vi "main.vi"() -> ()   [LabVIEW 2018]
uses:
  <vilib>/Platform/TimedLoop/XDataNode/XDataNode.xnode
  <vilib>/Platform/TimedLoop/XDataNode/nitl_modes.ctl
  <vilib>/Platform/TimedLoop/XDataNode/XDNodeRunTimeDep.lvlib
  <vilib>/Platform/TimedLoop/XDataNode/wakeup.ctl
  <vilib>/Platform/TimedLoop/XDataNode/timing_clust.ctl
  <vilib>/rvi/interface/nirviOpenFPGA/nirviOpenFPGA.xnode
  <vilib>/rvi/interface/nirviReadWriteControl/nirviReadWriteControl.xnode
  <vilib>/rvi/interface/Simulation/niFpgaSimulationCallBeginRW.vi
  <vilib>/rvi/errors/niLvFpgaAdjustHostInterfaceError.vi
  Labview_code/control6acater01.vi
  NiFpgaLv.dll
  <vilib>/Utility/error.llb/Error Cluster From Error Code.vi
  FPGA Bitfiles/Control 1.ctl
panel:
  out "Input Command":dbl[](array[numeric])
  out "now pwm":T1
  out "Finished delay inner loop":i32
  out "notEndmission":bool
  out "Finished delay":i32
  out "Good solution":bool
  out "length of each link":T2
  out "output PWM":cluster{dbl, dbl, dbl, dbl, dbl, dbl}
  in  "stop":T3
  # "StewHoward Platform"
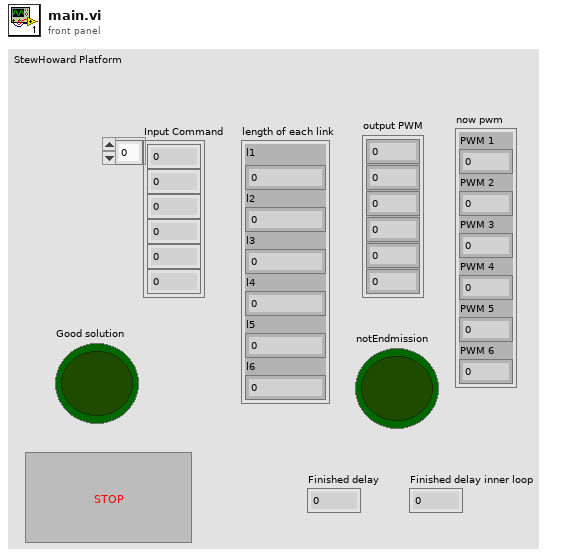
[diagram p1: front panel]
types:
  T1 = cluster{"PWM 1":dbl, "PWM 2":dbl, "PWM 3":dbl, "PWM 4":dbl, "PWM 5":dbl, "PWM 6":dbl}
  T2 = cluster{"l1":dbl, "l2":dbl, "l3":dbl, "l4":dbl, "l5":dbl, "l6":dbl}
  T3 = typedef "Control 1.ctl" = bool
  T4 = typedef "XDNodeRunTimeDep.lvlib/timing_clust.ctl" = cluster{"Expected End [f-1]":u64, "Actual End [f-1]":u64, "Finished Late? [f-1]":bool, "Expected End [i-1]":u64, "Actual End [i-1]":u64, "Finished Late? [i-1]":bool, "Expected Start [i]":u64, "Actual Start [i]":u64, "Expected Start [f]":u64, "Actual Start [f]":u64, "Source Name":string, "Structure Name":string, "Period":i64, "Deadline":i64, "Offset":i64, "Start":i64, "Priority":i32, "Timeout":i32, "Mode":T5, "Wakeup Reason":T6, "Error":errorcluster, "Source Type":string, "Secondary Source Type":string, "Global End Time":u64, "Global Start Time":u64, "Frame Duration":u64, "Iteration Duration":u64, "Assigned CPU":i32, "I/O Scan Engine Mode":u32}
  T5 = typedef "XDNodeRunTimeDep.lvlib/nitl_modes.ctl" = enum32{"No Change", "Process missed periods, maintain original phase", "Discard missed periods, maintain original phase", "Process missed periods, ignore original phase", "Discard missed periods, ignore original phase"}
  T6 = typedef "XDNodeRunTimeDep.lvlib/wakeup.ctl" = enum32{"Normal", "Aborted", "Asynchronous wakeup", "Timing source error", "Timed loop error", "Timeout"}
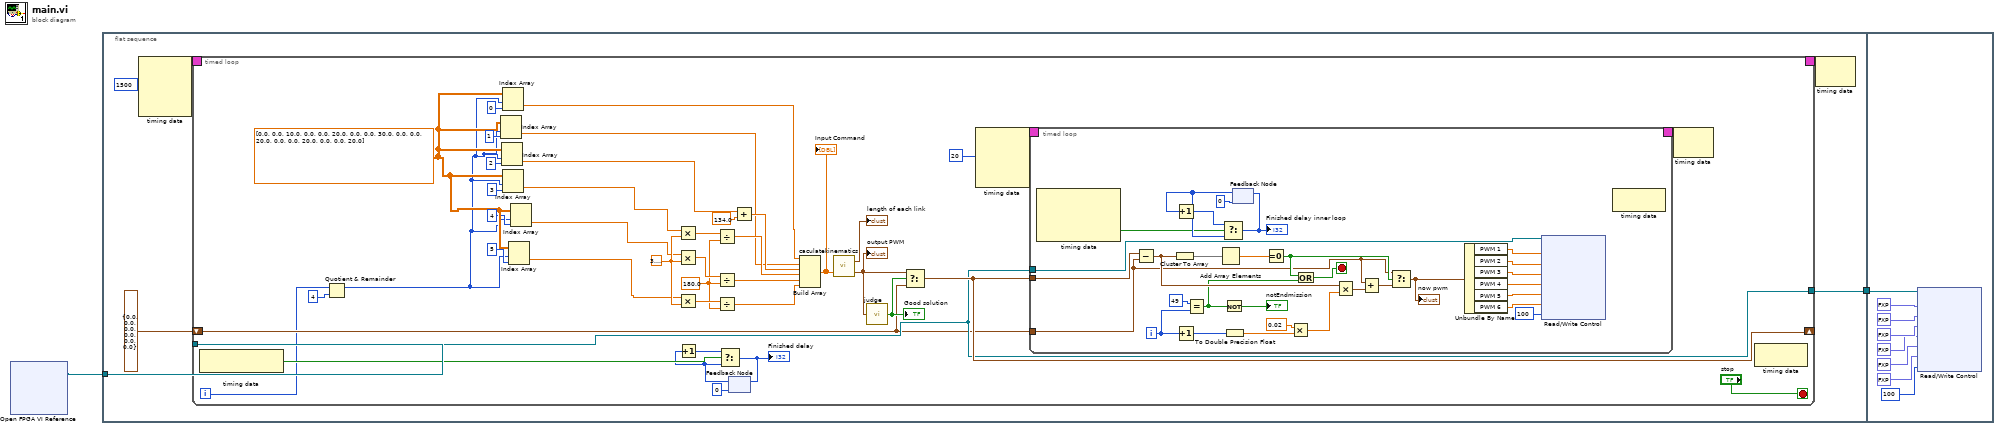
[diagram p0: block diagram]
diagram:
  n1 = xnode "Open FPGA VI Reference"() -> ("FPGA VI Reference Out"=w2:refnum<k20>)  [unwired: 2 in, 1 out]
  n2 = flat-sequence {
    tunnel: w2 -> [w8]
    tunnel: [w7] -> w1
    tunnel: w1 -> [w96]
    frame #0 {
      n3 = node-c288(i64 1500 ("Period")) -> (w6:T4)  [unwired: 3 in]
      n4 = timed-loop {
        tunnel: w8 -> [w38]
        shift-right: [w50] -> _
        shift-left: T1 {"PWM 1"=0.0, "PWM 2"=0.0, "PWM 3"=0.0, "PWM 4"=0.0, "PWM 5"=0.0, "PWM 6"=0.0} ("output PWM") -> [w25]
        tunnel: [w38] -> w7
        timing: w6 -> [_]
        timing-out: [_] -> w5
        i -> [w17]
        stop <- "stop" stop-if-true
        w24 = dbl[][] [[0.0, 0.0, 10.0], [0.0, 0.0, 20.0], [0.0, 0.0, 30.0], [0.0, 0.0, 20.0], [0.0, 0.0, 20.0], [0.0, 0.0, 20.0]]
        w43 = 180.0 ("y")
        w47 = 3.141592653589793
        n5 = node-c288() -> (w37:bool)  [unwired: 1 in]
        n6 = Quotient & Remainder(x=w17, y=4) -> (x-y*floor(x/y)=w15:i32)  [unwired: 1 out]
        n7 = Index Array(array=w24, index (row)=w15, index (col)=1 ("disabled index (col)")) -> (element=w10:dbl)
        n8 = Index Array(array=w24, index (row)=w15, index (col)=2 ("disabled index (col)")) -> (element=w11:dbl)
        n9 = Index Array(array=w24, index (row)=w15, index (col)=0 ("disabled index (col)")) -> (element=w9:dbl)
        n10 = Index Array(array=w24, index (row)=w15, index (col)=3 ("disabled index (col)")) -> (element=w14:dbl)
        n11 = Index Array(array=w24, index (row)=w15, index (col)=5 ("disabled index (col)")) -> (element=w12:dbl)
        n12 = Index Array(array=w24, index (row)=w15, index (col)=4 ("disabled index (col)")) -> (element=w13:dbl)
        n13 = Multiply(x=w14, y=w47) -> (x*y=w46:dbl)
        n14 = Multiply(x=w13, y=w47) -> (x*y=w45:dbl)
        n15 = Multiply(x=w12, y=w47) -> (x*y=w44:dbl)
        n16 = Divide(x=w46, y=w43) -> (x/y=w42:dbl)
        n17 = Divide(x=w45, y=w43) -> (x/y=w41:dbl)
        n18 = Divide(x=w44, y=w43) -> (x/y=w40:dbl)
        n19 = feedback #1(0) -> (w35:i32)
        n20 = Increment(x=w35) -> (x+1=w34:i32)
        n21 = Select(t=w34, s=w37, f=w35) -> (s? t:f=w33:i32)
        "Finished delay" <- w33
        n22 = feedback-in #1(w33) -> ()
        n23 = Add(x=w11, y=134.0) -> (x+y=w49:dbl)
        n24 = Build Array(w9, w10, w49, w42, w41, w40) -> (w28:dbl[])
        "Input Command" <- w28
        n25 = call "caculatekinematics.vi"("Input attitude array"=w28) -> ("output PWM"=w32:T1, "length of each link"=→"length of each link":T2)  [unwired: 1 in]
        "output PWM" <- w32
        n26 = call "judge.vi"("Cluster"=w32) -> ("logical AND"=w27:bool)
        "Good solution" <- w27
        n27 = Select(t=w32, s=w27, f=w25) -> (s? t:f=w50:T1)
        n28 = node-c288(i64 20 ("Period")) -> (w30:T4)  [unwired: 3 in]
        n29 = timed-loop {
          timing: w30 -> [_]
          timing-out: [_] -> w29
          tunnel: w50 -> [w52]
          tunnel: w38 -> [w81]
          tunnel: w25 -> [w51]
          i -> [w71]
          stop <- w55 stop-if-true
          n30 = node-c288() -> (w62:bool)  [unwired: 1 in, 3 out]
          n31 = Subtract(x=w52, y=w51) -> (x-y=w61:T1)
          n32 = Cluster To Array(cluster=w61) -> (array=w60:dbl[])
          n33 = Increment(x=w71) -> (x+1=w69:i32)
          n34 = Equal?(x=49, y=w71) -> (x = y?=w56:bool)
          n35 = Add Array Elements(numeric array=w60) -> (sum=w59:dbl)
          n36 = Not(x=w56) -> (.not. x?=→"notEndmission":bool)
          n37 = To Double Precision Float(number=w69) -> (double precision float=w70:dbl)
          n38 = feedback #2(0) -> (w64:i32)
          n39 = Increment(x=w64) -> (x+1=w65:i32)
          n40 = Select(t=w65, s=w62, f=w64) -> (s? t:f=w66:i32)
          "Finished delay inner loop" <- w66
          n41 = feedback-in #2(w66) -> ()
          n42 = Equal To 0?(x=w59) -> (x = 0?=w57:bool)
          n43 = Multiply(x=0.02, y=w70) -> (x*y=w67:dbl)
          n44 = Or(x=w57, y=w56) -> (x .or. y?=w55:bool)
          n45 = Multiply(x=w61, y=w67) -> (x*y=w54:T1)
          n46 = Add(x=w51, y=w54) -> (x+y=w53:T1)
          n47 = Select(t=w51, s=w57, f=w53) -> (s? t:f=w58:T1)
          "now pwm" <- w58
          n48 = Unbundle By Name(w58) -> ("PWM 1"=w80:dbl, "PWM 2"=w79:dbl, "PWM 3"=w78:dbl, "PWM 4"=w77:dbl, "PWM 5"=w76:dbl, "PWM 6"=w75:dbl)
          n49 = xnode "Read/Write Control"("FPGA VI Reference In"=w81, "Duty Cycle"=w80, "Duty Cycle 2"=w79, "Duty Cycle 3"=w78, "Duty Cycle 4"=w77, "Duty Cycle 5"=w76, "Duty Cycle 6"=w75, "Period (Ticks)"=u32 100) -> ()  [unwired: 1 in, 2 out]
          n50 = node-c288() -> ()  [unwired: 1 in, 1 out]
        }
        n51 = node-c288(w29) -> ()  [unwired: 1 out]
        n52 = node-c288() -> ()  [unwired: 1 in, 1 out]
      }
      n53 = node-c288(w5) -> ()  [unwired: 1 out]
    }
    frame #1 {
      n54 = xnode "Read/Write Control"("FPGA VI Reference In"=w96, "Duty Cycle"=fxp<+,32,0> 0.0, "Duty Cycle 2"=fxp<+,32,0> 0.0, "Duty Cycle 3"=fxp<+,32,0> 0.0, "Duty Cycle 4"=fxp<+,32,0> 0.0, "Duty Cycle 5"=fxp<+,32,0> 0.0, "Duty Cycle 6"=fxp<+,32,0> 0.0, "Period (Ticks)"=u32 100) -> ()  [unwired: 1 in, 2 out]
    }
  }
